vi "display.vi"(8 "error in (no error)":errorcluster, 11 "MallardDuck in":refnum<class "MallardDuck.lvclass">) -> (0 "error out":errorcluster, 2 "State":string, 3 "MallardDuck out":refnum<class "MallardDuck.lvclass">)   [LabVIEW 2013, in "MallardDuck.lvclass"]
uses:
  MallardDuck.lvclass
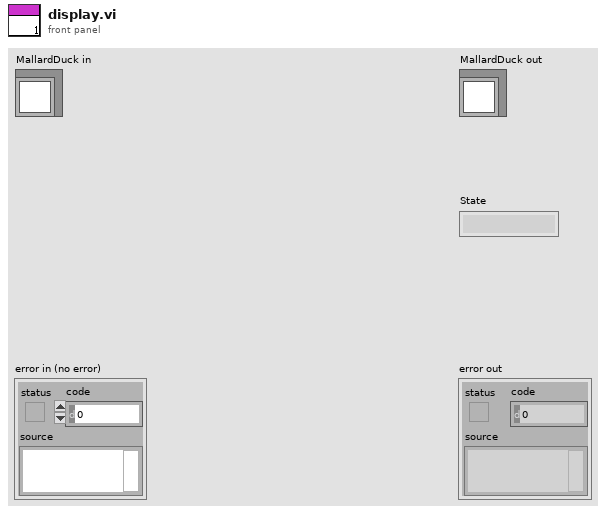
[diagram p1: front panel]
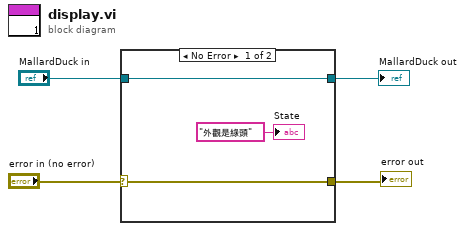
[diagram p0: block diagram]
diagram:
  n1 = case shown="No Error" "error in (no error)" {
    selector: "error in (no error)" -> [w7 w9]
    tunnel: [w7 w9] -> w3
    tunnel: [w6 w8] -> w2
    tunnel: "MallardDuck in" -> [w6 w8]
    frame No Error {
      "State" <- "外觀是綠頭" ("State")
    }
    frame Error {
    }
  }
  "error out" <- w3
  "MallardDuck out" <- w2
